vi "battery.vi"(1 "error IO in":errorcluster) -> (0 "error IO":errorcluster)   [LabVIEW 2013]
panel:
  # "- Battery fill state\n- assumed operation time"
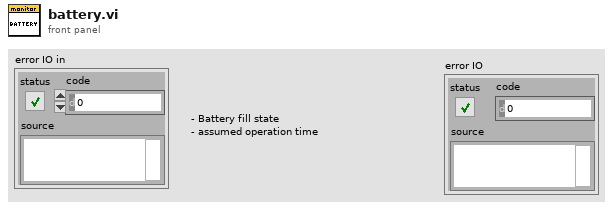
[diagram p1: front panel]
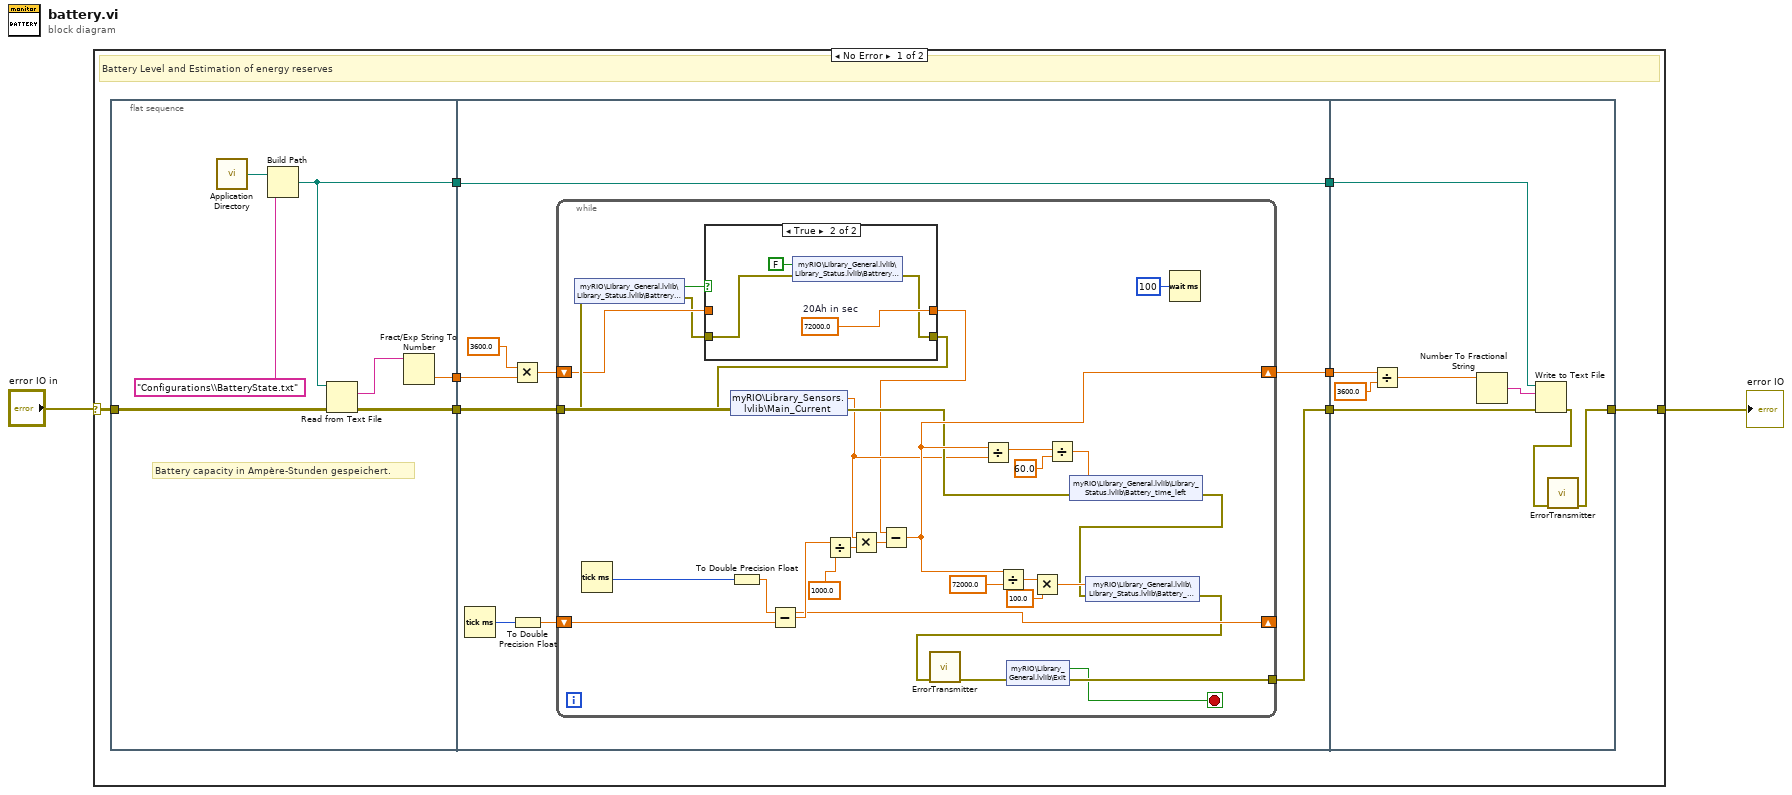
[diagram p0: block diagram]
diagram:
  n1 = case shown="No Error" "error IO in" {
    selector: "error IO in" -> [w9 w70]
    tunnel: [w10 w70] -> w2
    frame No Error {
      # "Battery Level and Estimation of energy reserves"
      n2 = flat-sequence {
        tunnel: w9 -> [w17]
        tunnel: [w16] -> w8
        tunnel: [w11] -> w7
        tunnel: [w13] -> w5
        tunnel: w8 -> [w26]
        tunnel: w7 -> [w20]
        tunnel: [w23] -> w6
        tunnel: w5 -> [w23]
        tunnel: [w22] -> w4
        tunnel: [w18] -> w3
        tunnel: [w64] -> w10
        tunnel: w6 -> [w68]
        tunnel: w4 -> [w67]
        tunnel: w3 -> [w69]
        frame #0 {
          # "Battery capacity in Ampère-Stunden gespeichert."
          n3 = call <vilib>:"Application Directory.vi"() -> ("Application Directory"=w14:path)
          n4 = Build Path(base path=w14, name or relative path="Configurations\\BatteryState.txt" ("string")) -> (appended path=w13:path)
          n5 = Read from Text File(file (use dialog)=w13, error in=w17) -> (text=w12:string, error out=w16:errorcluster)  [unwired: 2 in, 2 out]
          n6 = Fract/Exp String To Number(string=w12) -> (number=w11:dbl)  [unwired: 3 in, 1 out]
        }
        frame #1 {
          n7 = Tick Count (ms)() -> (millisecond timer value=w25:u32)
          n8 = Multiply(x=3600.0, y=w20) -> (x*y=w21:dbl)
          n9 = To Double Precision Float(number=w25) -> (double precision float=w24:dbl)
          n10 = while {
            shift-right: [w46] -> w22
            shift-left: w21 -> [w30]
            shift-right: [w47] -> _
            shift-left: w24 -> [w52]
            tunnel: w26 -> [w32]
            tunnel: [w43] -> w18
            stop <- w38 stop-if-true
            n11 = shared-variable "myRIO\\Library_General.lvlib\\Library_Status.lvlib\\Battrery_Full"(error in=w32) -> (w33:bool, error out=w29:errorcluster)
            n12 = Tick Count (ms)() -> (millisecond timer value=w48:u32)
            n13 = case shown="True" w33 {
              tunnel: [w57 w61] -> w31
              tunnel: w30 -> [w57 _]
              tunnel: w29 -> [w56 w59]
              tunnel: [w56 w58] -> w28
              frame False {
              }
              frame True {
                w61 = 72000.0  # 20Ah in sec
                n14 = shared-variable "myRIO\\Library_General.lvlib\\Library_Status.lvlib\\Battrery_Full"(FALSE ("Battrery_Full"), error in=w59) -> (error out=w58:errorcluster)
              }
            }
            n15 = shared-variable "myRIO\\Library_Sensors.lvlib\\Main_Current"(error in=w28) -> (w37:dbl, error out=w39:errorcluster)
            n16 = To Double Precision Float(number=w48) -> (double precision float=w47:dbl)
            n17 = Subtract(x=w47, y=w52) -> (x-y=w49:dbl)
            n18 = Divide(x=w49, y=1000.0) -> (x/y=w50:dbl)
            n19 = Multiply(x=w37, y=w50) -> (x*y=w51:dbl)
            n20 = Subtract(x=w31, y=w51) -> (x-y=w46:dbl)
            n21 = Divide(x=w46, y=w37) -> (x/y=w45:dbl)
            n22 = Divide(x=w46, y=72000.0) -> (x/y=w54:dbl)
            n23 = Multiply(x=w54, y=100.0) -> (x*y=w40:dbl)
            n24 = Divide(x=w45, y=60.0) -> (x/y=w41:dbl)
            n25 = shared-variable "myRIO\\Library_General.lvlib\\Library_Status.lvlib\\Battery_time_left"(w41, error in=w39) -> (error out=w36:errorcluster)
            n26 = shared-variable "myRIO\\Library_General.lvlib\\Library_Status.lvlib\\Battery_Level"(w40, error in=w36) -> (error out=w34:errorcluster)
            n27 = call "ErrorTransmitter.vi"("Error In"=w34) -> ("Error Out"=w35:errorcluster)  [unwired: 10 in]
            n28 = shared-variable "myRIO\\Library_General.lvlib\\Exit"(error in=w35) -> (w38:bool, error out=w43:errorcluster)
            n29 = Wait (ms)(milliseconds to wait=u32 100) -> ()  [unwired: 1 out]
          }
        }
        frame #2 {
          n30 = Divide(x=w67, y=3600.0) -> (x/y=w63:dbl)
          n31 = Number To Fractional String(number=w63) -> (F-format string=w62:string)  [unwired: 3 in]
          n32 = Write to Text File(file (use dialog)=w68, text=w62, error in=w69) -> (error out=w65:errorcluster)  [unwired: 1 in, 2 out]
          n33 = call "ErrorTransmitter.vi"("Error In"=w65) -> ("Error Out"=w64:errorcluster)  [unwired: 10 in]
        }
      }
    }
    frame Error {
    }
  }
  "error IO" <- w2
